vi "classes.vi"(0 "HGF_Factory":refnum<class "HGF_DeviceBaseFactory.lvclass">, 1 "className":string, 5 "error in (no error)":errorcluster) -> (14 "HGF_Factory dup":refnum<class "HGF_DeviceBaseFactory.lvclass">, 16 "Object":refnum<class>, 19 "error out":errorcluster)   [LabVIEW 2014, in "HGF_DeviceBaseClasses.lvlib" / "HGF_DeviceBaseFactory.lvclass"]
doc: "This dynamaic dispatch VI contains constant objects of all classes that can be produced by HGF_Factory.\nClass has to be defined by name. \n\nOptionally, you can also specifiy a Class Path String instead, but you have to make sure that all dependencies are available.\n\nChild classes have to override it to define additional classes."
uses:
  HGF_DeviceBaseFactory.lvclass
  HGF_DeviceVisitor/HGF_Device_ErrorQuery/HGF_Device_ErrorQuery.lvclass
  HGF_DeviceVisitor/HGF_Device_IDN/HGF_Device_IDN.lvclass
  HGF_DeviceVisitor/HGF_Device_Reset/HGF_Device_Reset.lvclass
  HGF_DeviceVisitor/HGF_Device_SelfTest/HGF_Device_SelfTest.lvclass
  HGF_BaseClasses/HGF_Factory/HGF_Factory.lvclass
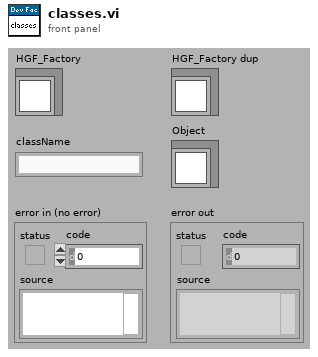
[diagram p1: front panel]
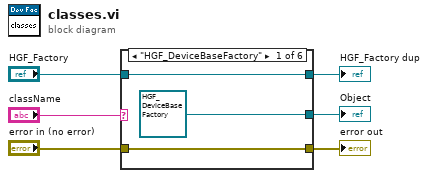
[diagram p0: block diagram]
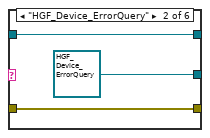
[diagram p2: hidden frame]
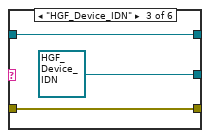
[diagram p3: hidden frame]
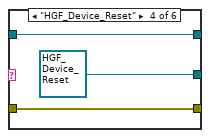
[diagram p4: hidden frame]
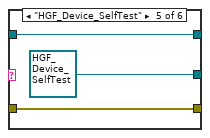
[diagram p5: hidden frame]
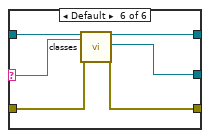
[diagram p6: hidden frame]
diagram:
  n1 = case shown="\"HGF_DeviceBaseFactory\"" "className" {
    selector: "className" -> [_ _ _ _ _ w26]
    tunnel: [refnum<class "HGF_DeviceBaseFactory.lvclass"> refnum ("HGF_DeviceBaseClasses.lvlib:HGF_DeviceBaseFactory.lvclass") refnum<class "HGF_Device_ErrorQuery.lvclass"> refnum ("HGF_DeviceBaseClasses.lvlib:HGF_Device_ErrorQuery.lvclass") refnum<class "HGF_Device_IDN.lvclass"> refnum ("HGF_DeviceBaseClasses.lvlib:HGF_Device_IDN.lvclass") refnum<class "HGF_Device_Reset.lvclass"> refnum ("HGF_DeviceBaseClasses.lvlib:HGF_Device_Reset.lvclass") refnum<class "HGF_Device_SelfTest.lvclass"> refnum ("HGF_DeviceBaseClasses.lvlib:HGF_Device_SelfTest.lvclass") w27] -> w3
    tunnel: "error in (no error)" -> [w8 w11 w13 w17 w20 w23]
    tunnel: [w8 w11 w13 w17 w20 w22] -> w5
    tunnel: "HGF_Factory" -> [w7 w10 w14 w16 w19 w25]
    tunnel: [w7 w10 w14 w16 w19 w24] -> w1
    frame "HGF_DeviceBaseFactory" {
    }
    frame "HGF_Device_ErrorQuery" {
    }
    frame "HGF_Device_IDN" {
    }
    frame "HGF_Device_Reset" {
    }
    frame "HGF_Device_SelfTest" {
    }
    frame Default {
      n2 = call-parent "classes.vi"("HGF_Factory"=w25, "className"=w26, "error in (no error)"=w23) -> ("HGF_Factory dup"=w24:refnum<class "HGF_DeviceBaseFactory.lvclass">, "Object"=w27:refnum<class>, "error out"=w22:errorcluster)  [unwired: 14 out]
    }
  }
  "error out" <- w5
  "HGF_Factory dup" <- w1
  "Object" <- w3
